vi "cam take photo.vi"(7 "error in":errorcluster) -> (20 "Image Out":T2(plugin-control), 21 "Session Out":T1, 27 "error out":errorcluster)   [LabVIEW 2019]
doc: "Creates, and edits acquisitions using the NI Vision Acquisition Express VI.\n\nThe NI Vision Acquisition Wizard is launched by placing the Express VI on the block diagram. Select an acquisition source and configure an acquisition using NI-IMAQ, NI-IMAQdx, or simulate an acquisition by reading an AVI or image files from a folder. After an acquisition is configured, select controls and indicators to be able to programmatically set in LabVIEW. Double-click the Vision Acquisition Express VI to edit the acquisition.\n\nNote: Any images created by the Express VI need to be disposed after use. Use the IMAQ Dispose.vi to cleanup the images output by the Express VI when they are no longer needed."
uses:
  <vilib>/userDefined/High Color/IMAQdx.ctl
  <vilib>/vision/driver/NI_Vision_Acquisition_Software.lvlib
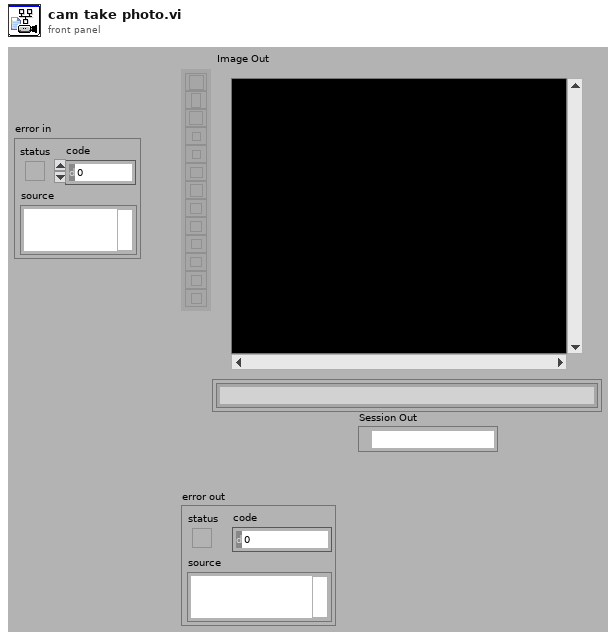
[diagram p1: front panel]
types:
  T1 = typedef "IMAQdx.ctl" = refnum<k21>
  T2 = typedef "IMAQ Image.ctl" = refnum<image>
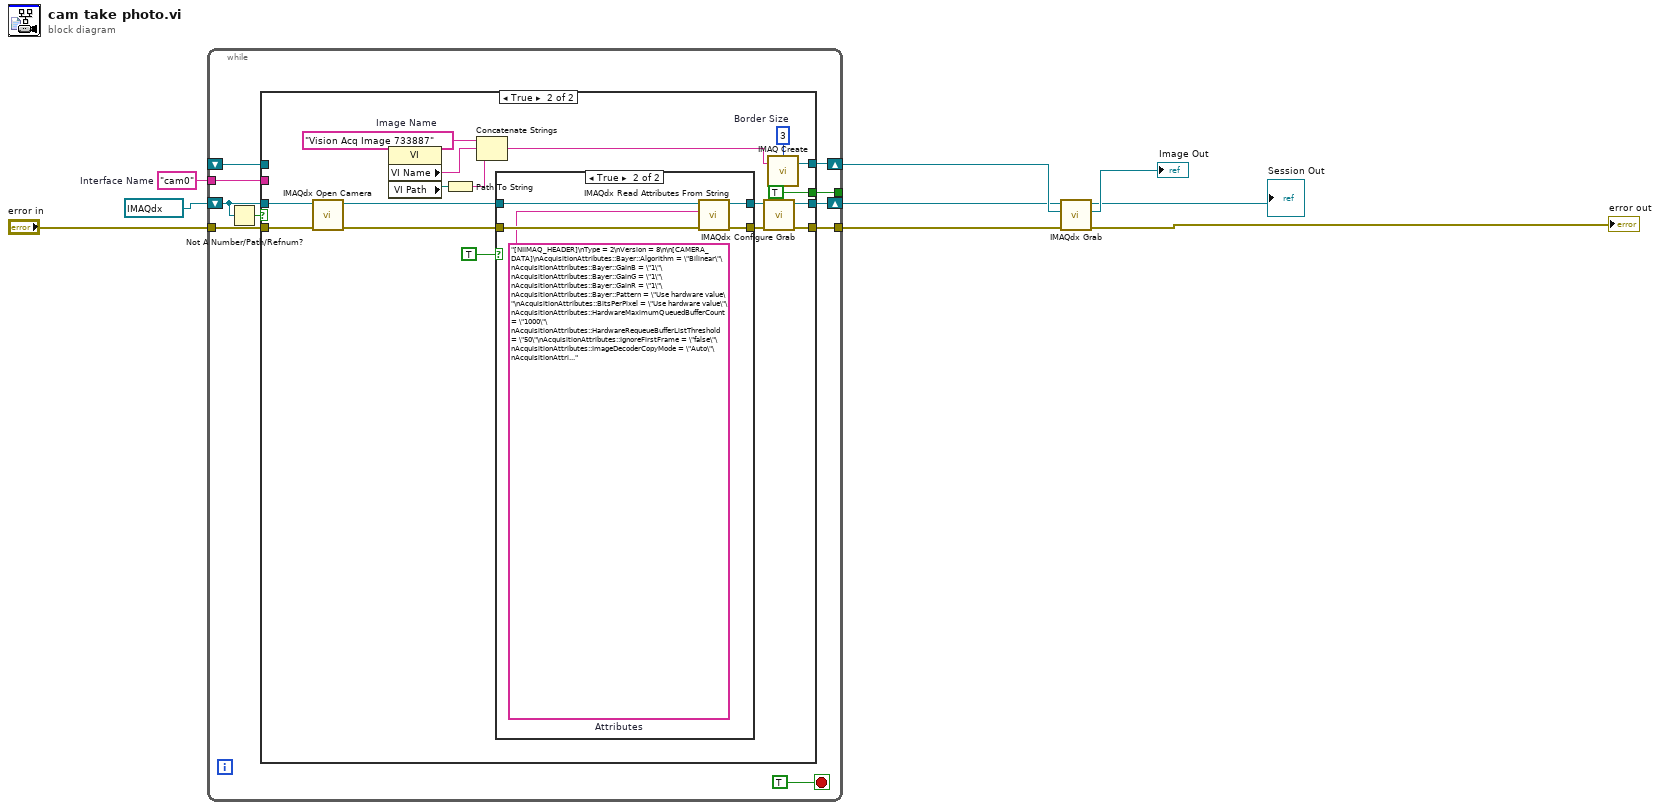
[diagram p0: block diagram]
diagram:
  w7 = "cam0"  # Interface Name
  n1 = while "While Loop_template0" {
    shift-right: [w19] -> w4
    shift-left: T1 "cam0" ("Session Out") -> [w12]
    tunnel: [w18] -> w8
    tunnel: "error in" -> [w17]
    shift-right: [w15] -> w5
    shift-left: _ -> [w14]
    tunnel: w7 -> [w13]
    tunnel: [w10] -> _
    stop <- TRUE ("_template0") stop-if-true
    n2 = Not A Number/Path/Refnum?(number/path/refnum=w12) -> (NaN/Path/Refnum?=w11:bool)
    n3 = case "Case Structure_template0" shown="True" w11 {
      tunnel: [w22 w38] -> w19
      tunnel: w12 -> [w22 w23]
      tunnel: [w21 w37] -> w18
      tunnel: w17 -> [w21 w39]
      tunnel: [w20 w36] -> w15
      tunnel: w14 -> [w20 _]
      tunnel: w13 -> [_ _]
      tunnel: [_ TRUE] -> w10
      frame False {
      }
      frame True {
        w24 = 3  # Border Size
        w31 = "Vision Acq Image 733887"  # Image Name
        n4 = call <vilib>:"IMAQdx Open Camera.vi"("error in"=w39, "Session In"=w23) -> ("error out"=w29:errorcluster, "Session Out"=w30:T1)  [unwired: 1 in, 7 out]
        n5 = property class="VI"() -> ("VI Name"=w34:string, "VI Path"=w35:path)  [unwired: 2 in, 2 out]
        n6 = Path To String(path=w35) -> (string=w33:string)
        n7 = Concatenate Strings(w31, w34, w33) -> (w32:string)
        n8 = case shown="True" TRUE ("Init Attributes") {
          tunnel: w30 -> [w41 w46]
          tunnel: w29 -> [w40 w45]
          tunnel: [w41 w43] -> w28
          tunnel: [w40 w42] -> w27
          frame False {
          }
          frame True {
            w44 = "[NIIMAQ_HEADER]\nType = 2\nVersion = 8\n\n[CAMERA_DATA]\nAcquisitionAttributes::Bayer::Algorithm = \"Bilinear\"\nAcquisitionAttributes::Bayer::GainB = \"1\"\nAcquisitionAttributes::Bayer::GainG = \"1\"\nAcquisitionAttributes::Bayer::GainR = \"1\"\nAcquisitionAttributes::Bayer::Pattern = \"Use hardware value\"\nAcquisitionAttributes::BitsPerPixel = \"Use hardware value\"\nAcquisitionAttributes::HardwareMaximumQueuedBufferCount = \"1000\"\nAcquisitionAttributes::HardwareRequeueBufferListThreshold = \"50\"\nAcquisitionAttributes::IgnoreFirstFrame = \"false\"\nAcquisitionAttributes::ImageDecoderCopyMode = \"Auto\"\nAcquisitionAttributes::OutputImageType = \"Auto\"\nAcquisitionAttributes::OverwriteMode = \"Get Newest\"\nAcquisitionAttributes::PixelSignedness = \"Use hardware value\"\nAcquisitionAttributes::ReceiveTimestampMode = \"None\"\nAcquisitionAttributes::ShiftPixelBits = \"false\"\nAcquisitionAttributes::SwapPixelBytes = \"false\"\nAcquisitionAttributes::Timeout = \"5000\"\nAcquisitionAttributes::VideoMode = \"160 x 120 YUY 2 30.00 fps\"\nCameraAttributes::BacklightCompensation::Mode = \"Manual\"\nCameraAttributes::BacklightCompensation::Value = \"10\"\nCameraAttributes::Brightness::Mode = \"Manual\"\nCameraAttributes::Brightness::Value = \"133\"\nCameraAttributes::Contrast::Mode = \"Manual\"\nCameraAttributes::Contrast::Value = \"5\"\nCameraAttributes::Exposure::Mode = \"Manual\"\nCameraAttributes::Exposure::Value = \"156\"\nCameraAttributes::Focus::Mode = \"Auto\"\nCameraAttributes::Pan::Mode = \"Manual\"\nCameraAttributes::Pan::Value = \"0\"\nCameraAttributes::PowerLineFrequency::Mode = \"60Hz\"\nCameraAttributes::Saturation::Mode = \"Manual\"\nCameraAttributes::Saturation::Value = \"83\"\nCameraAttributes::Sharpness::Mode = \"Manual\"\nCameraAttributes::Sharpness::Value = \"25\"\nCameraAttributes::Tilt::Mode = \"Manual\"\nCameraAttributes::Tilt::Value = \"0\"\nCameraAttributes::WhiteBalance::Mode = \"Manual\"\nCameraAttributes::WhiteBalance::Value = \"4575\"\nCameraAttributes::Zoom::Mode = \"Manual\"\nCameraAttributes::Zoom::Value = \"0\"\n"  # Attributes
            n9 = call <vilib>:"IMAQdx Read Attributes From String.vi"("error in"=w45, "Attributes String In"=w44, "Session In"=w46) -> ("error out"=w42:errorcluster, "Session Out"=w43:T1)  [unwired: 7 out]
          }
        }
        n10 = call <vilib>:"IMAQdx Configure Grab.vi"("error in"=w27, "Session In"=w28) -> ("error out"=w37:errorcluster, "Session Out"=w38:T1)  [unwired: 1 in, 7 out]
        n11 = call "IMAQ Create"("Border Size"=w24, "Image Name"=w32) -> ("New Image"=w36:T2)  [unwired: 2 in, 2 out]
      }
    }
  }
  n12 = call <vilib>:"IMAQdx Grab.vi"("error in"=w8, "Image In"=w5, "Session In"=w4) -> ("error out"=→"error out":errorcluster, "Image Out"=→"Image Out":T2, "Session Out"=→"Session Out":T1)  [unwired: 1 in, 5 out]
